vi "AO tester.vi"() -> ()   [LabVIEW 2013]
uses:
  Controls/FPGA Nain State.ctl
  <vilib>/Platform/TimedLoop/XDataNode/timing_clust.ctl
  <vilib>/Platform/TimedLoop/XDataNode/nitl_modes.ctl
  <vilib>/Platform/TimedLoop/XDataNode/wakeup.ctl
  Controls/Algorithm State.ctl
  <vilib>/rvi/Emulation/niFpgaSctlEmulationGetInTimedLoop.vi
  <vilib>/rvi/Emulation/niFpgaEmulationReportErrorSimple.vi
  <vilib>/rvi/Emulation/niFpgaGetClockAttributes.vi
  <vilib>/rvi/Emulation/niFpgaCriticalErrorInLSC.vi
  <vilib>/rvi/FIFO/Fifo_Resource/nirvififoEmulationReadFpgaImpl.vi
  <vilib>/rvi/DataTransferAndStorage/Container/Common/niFpgaContainerGetUniqueNameForEmu.vi
  <vilib>/rvi/interface/RandomDataEmulation/nirviRandomDataFPGAFIFO.vi
  <vilib>/rvi/interface/RandomDataEmulation/niFpgaRandomDataHandleErrors.vi
  <vilib>/rvi/eio/common/nirviEmuTemplateMethod_errors.vi
  <vilib>/rvi/FIFO/Fifo_Resource/nirvififoEmulationWriteFpgaImpl.vi
  LIDAR V2 Globals.vi
  <vilib>/rvi/Emulation/niFpgaProcessEmulError.vi
  <vilib>/Platform/TimedLoop/XDataNode/XDataNode.xnode
  <vilib>/rvi/DataTransferAndStorage/Container/XNode/niFpgaContainer.xnode
  <vilib>/rvi/FIFO/Fifo_Resource/nirvififoEmulationRead.vi
  <vilib>/rvi/interface/RandomDataEmulation/nirviRandomDataFpgaReadWriteTemplate.vi
  <vilib>/eio/EIONode/EIONode.xnode
  <vilib>/rvi/FIFO/Fifo_Resource/nirvififoEmulationWrite.vi
  <vilib>/Platform/TimedLoop/XDataNode/XDNodeRunTimeDep.lvlib
panel:
  out "EndOfPulseGen":bool
  in  "SingleFrame":bool
  out "Port1":u8 format="%.0b"
  out "Port1Bit5":bool
  out "Port1Bit4":bool
  out "Port0":u8 format="%.0b"
  in  "PFI2":bool
  in  "PFI3":bool
  in  "WaitForPulseEndDelay":u8=3
  in  "ActiveLedIndexDeb":u16
  in  "LedScanDebEn":bool
  in  "NoOfLeds":u16=320
  out "LedAddress":u16
  in  "SamplingEnable":bool
  out "MainState":T1
  in  "PulseEndClck":u8=3
  in  "PulseWaitClck":u8=40
  out "SimOut":i16
  out "PulseIndex":i16
  in  "PulsePerLed":i16=199
  in  "MemSel":bool
  out "ActiveLedIndex":u16
  in  "SampPerPulse":u8=100
  out "PulseEnd":bool
  out "Timeouts":u16
  in  "SPI Device":u8
  out "AI":i16
  in  "EnAI":bool
  in  "User Command Commit":bool
  in  "User Command":u8
  out "User Command Idle":bool
  out "User Command Status":u8
  in  "User Data 0":u8
  in  "User Data 1":u8
  out "User Error":bool
  out "Configured?":bool
  out "PLL Locked":bool
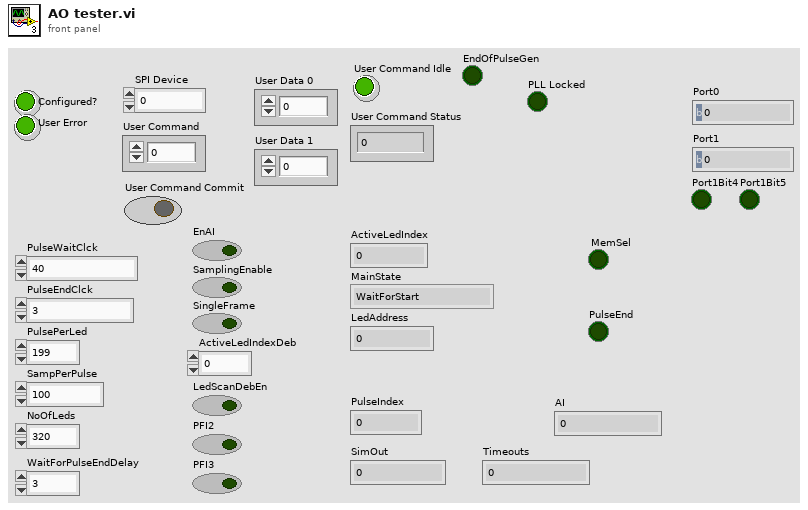
[diagram p1: front panel]
types:
  T1 = typedef "FPGA Nain State.ctl" = enum16{"WaitForStart", "SetProcParams", "SelectActiveLed", "WaitForPulseGenEnd", "ActivatePulse", "WaitForPulseEnd", "WaitForAlgoStart", "SingleCycleEnd"}
  T2 = typedef "XDNodeRunTimeDep.lvlib/timing_clust.ctl" = cluster{"Expected End [f-1]":u64, "Actual End [f-1]":u64, "Finished Late? [f-1]":bool, "Expected End [i-1]":u64, "Actual End [i-1]":u64, "Finished Late? [i-1]":bool, "Expected Start [i]":u64, "Actual Start [i]":u64, "Expected Start [f]":u64, "Actual Start [f]":u64, "Source Name":string, "Structure Name":string, "Period":i64, "Deadline":i64, "Offset":i64, "Start":i64, "Priority":i32, "Timeout":i32, "Mode":T3, "Wakeup Reason":T4, "Error":errorcluster, "Source Type":string, "Secondary Source Type":string, "Global End Time":u64, "Global Start Time":u64, "Frame Duration":u64, "Iteration Duration":u64, "Assigned CPU":i32, "I/O Scan Engine Mode":u32}
  T3 = typedef "XDNodeRunTimeDep.lvlib/nitl_modes.ctl" = enum32{"No Change", "Process missed periods, maintain original phase", "Discard missed periods, maintain original phase", "Process missed periods, ignore original phase", "Discard missed periods, ignore original phase"}
  T4 = typedef "XDNodeRunTimeDep.lvlib/wakeup.ctl" = enum32{"Normal", "Aborted", "Asynchronous wakeup", "Timing source error", "Timed loop error", "Timeout"}
  T5 = typedef "Algorithm State.ctl" = enum16{"WaitForStart", "GetNextSignalElement", "WaitForNextSignalElem", "MultWithSinc", "CalcMax"}
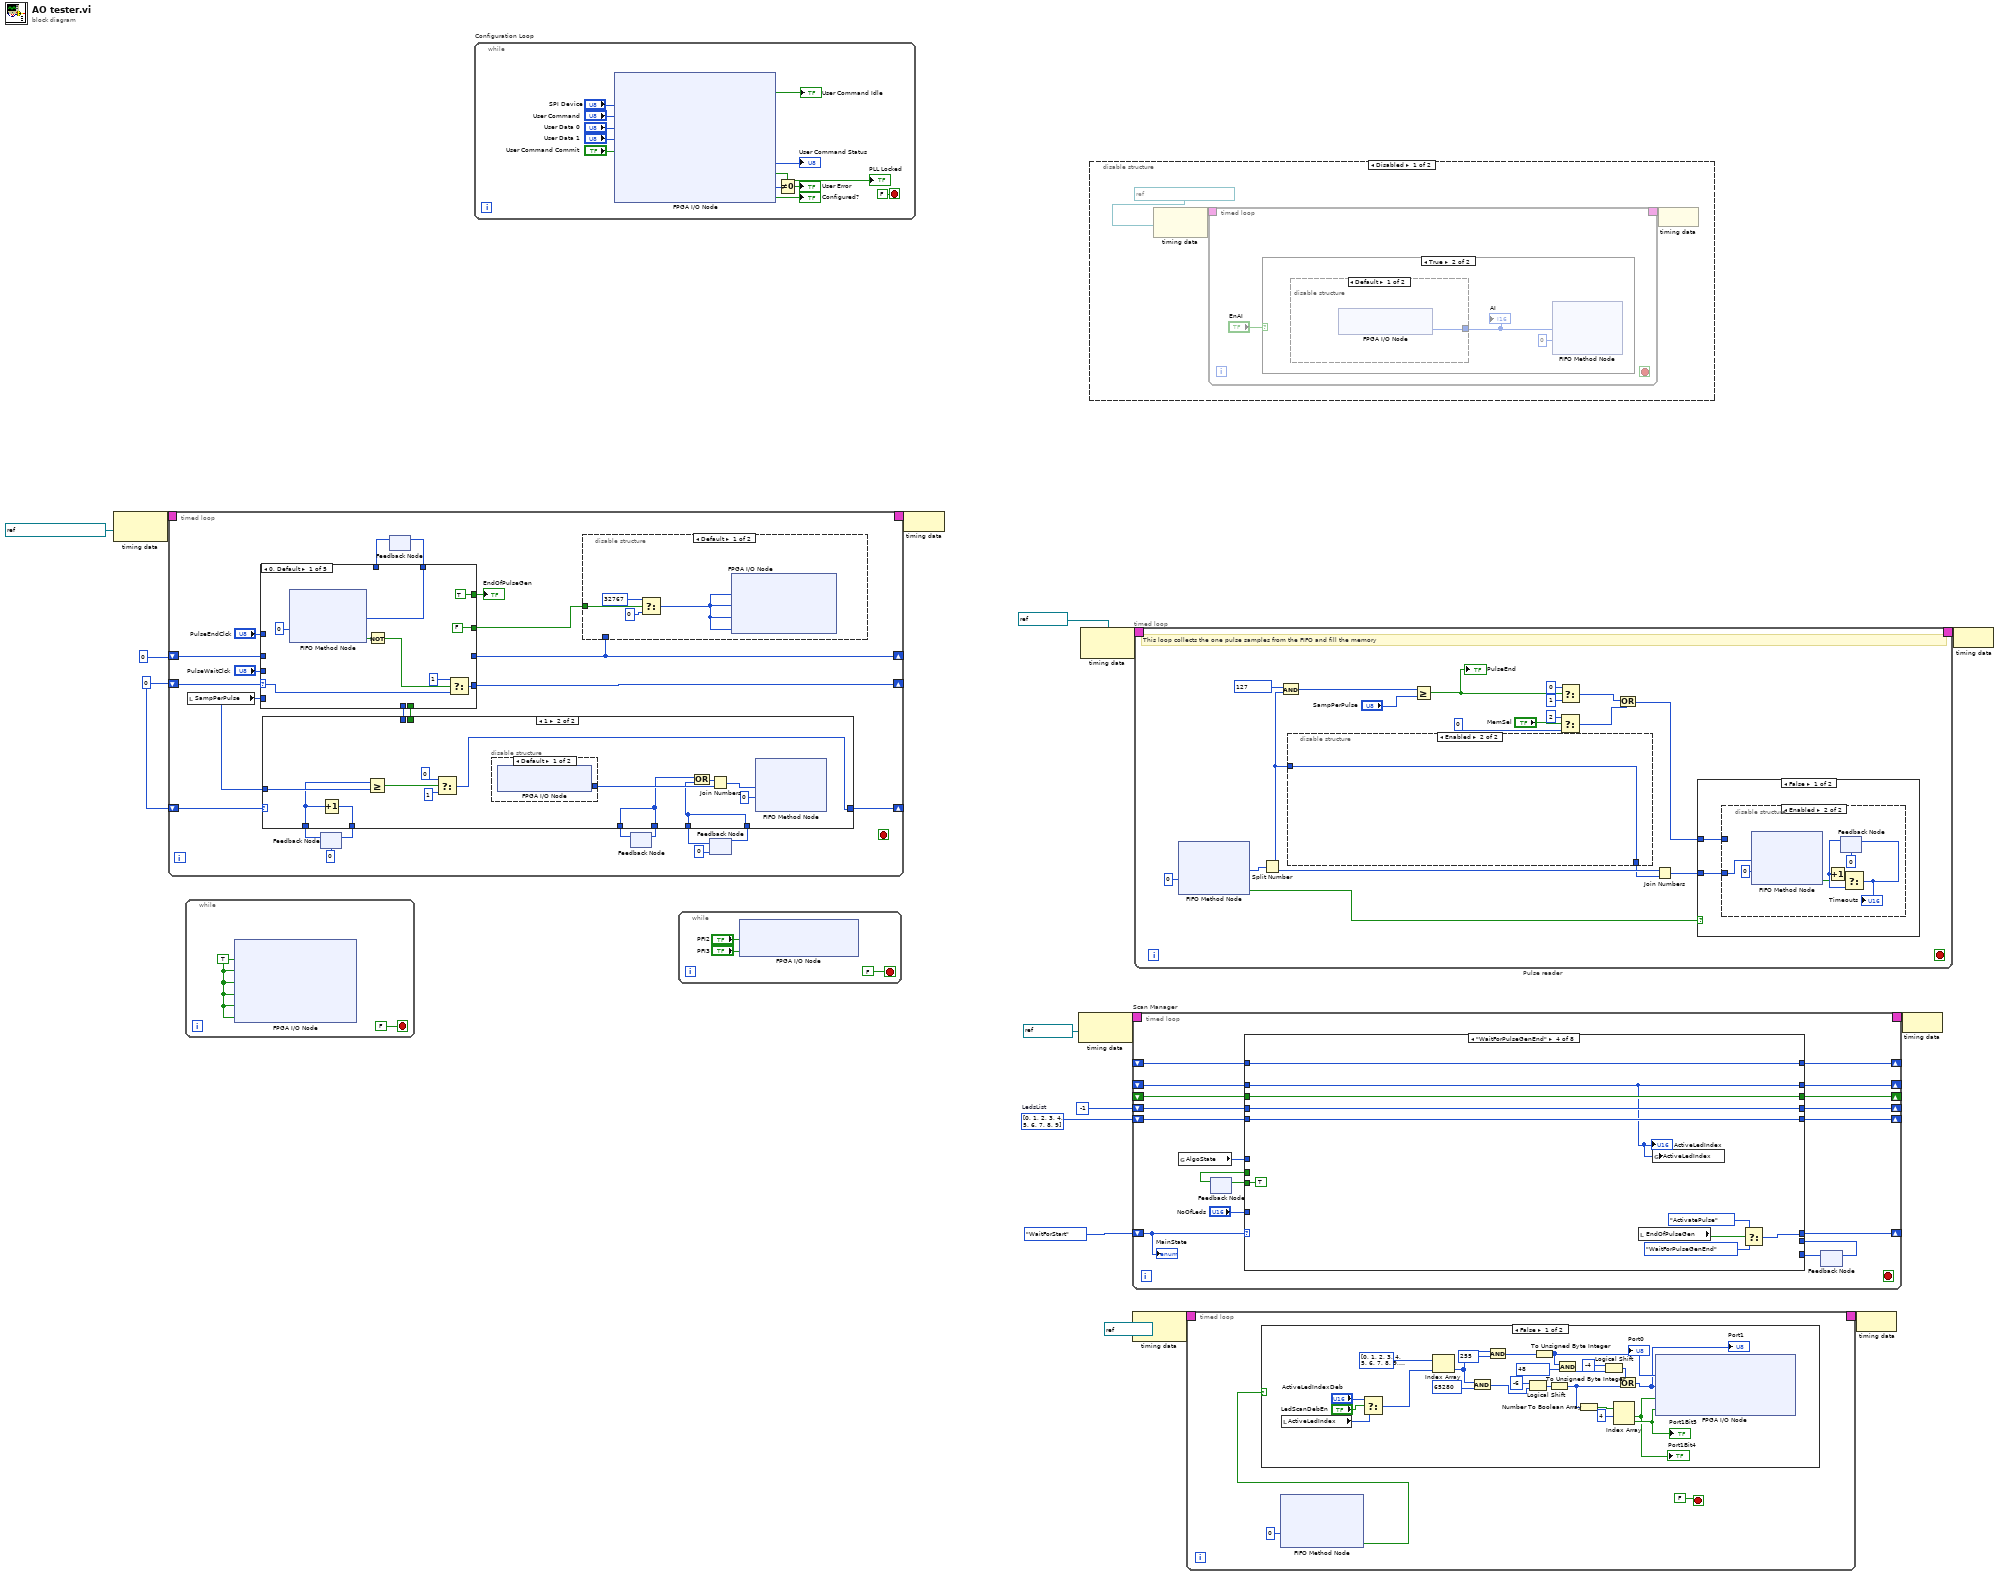
[diagram p0: block diagram]
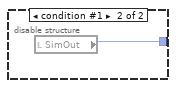
[diagram p3: hidden frame]
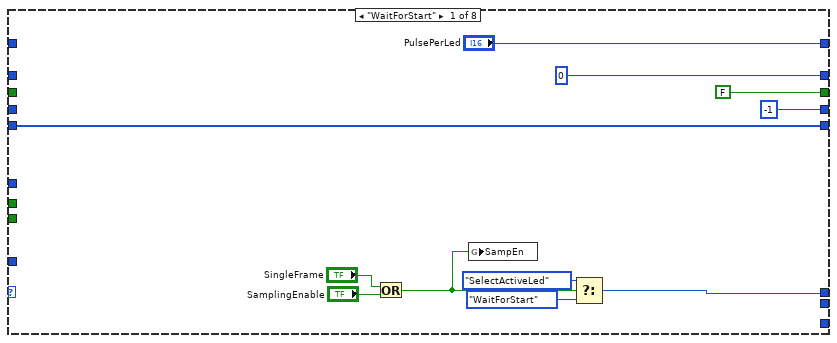
[diagram p6: hidden frame]
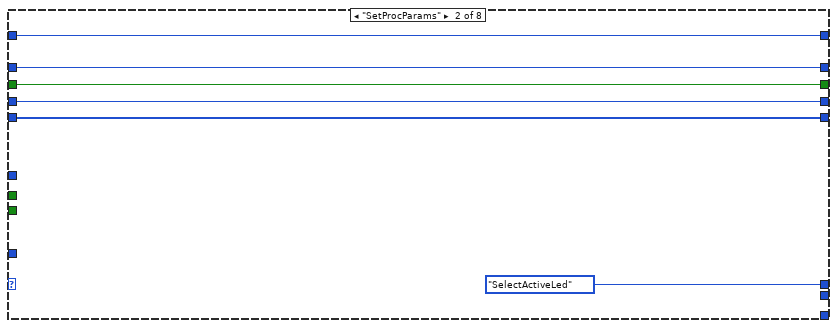
[diagram p7: hidden frame]
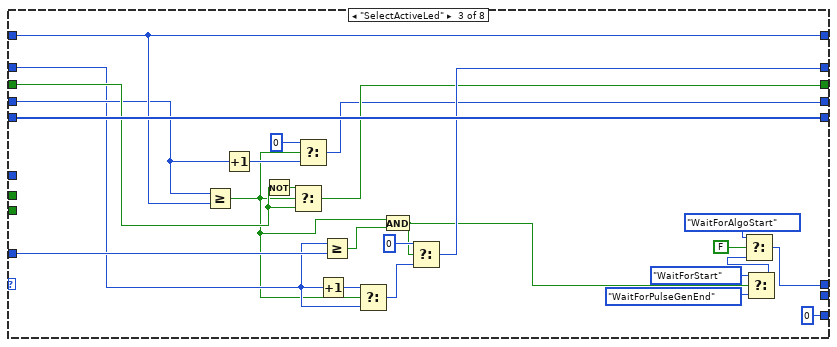
[diagram p8: hidden frame]
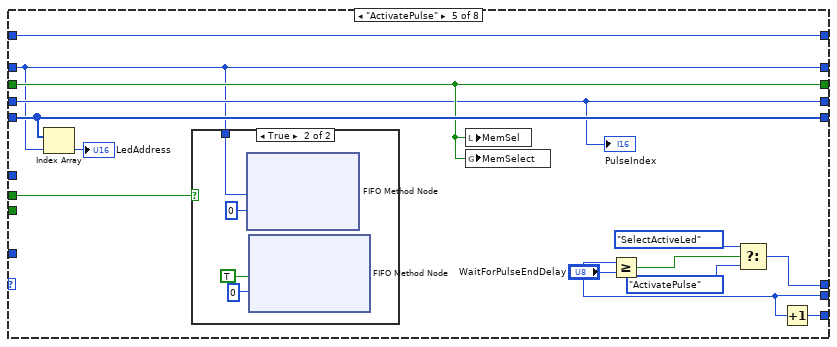
[diagram p9: hidden frame]
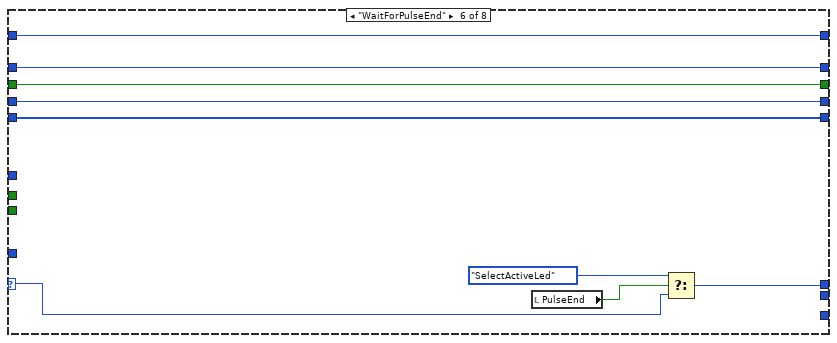
[diagram p11: hidden frame]
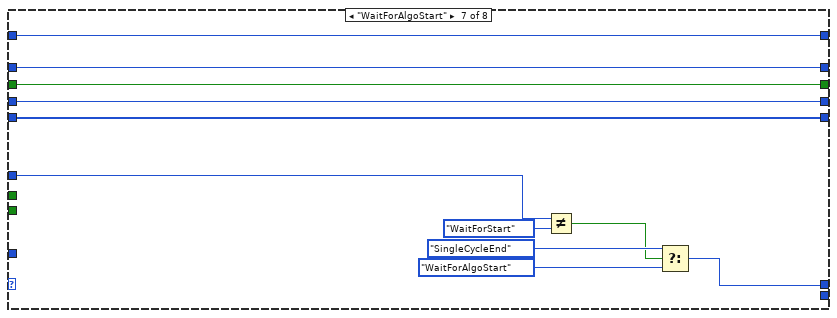
[diagram p12: hidden frame]
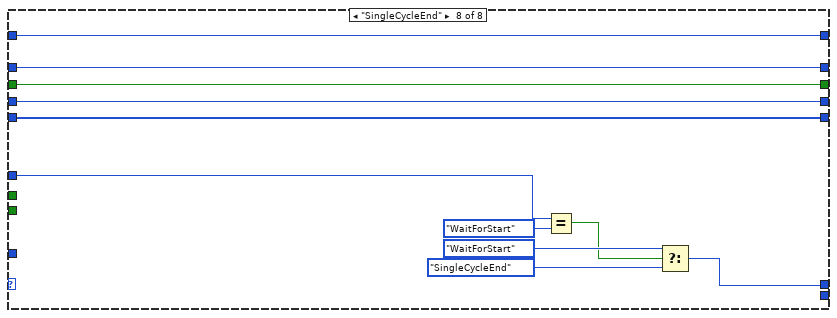
[diagram p13: hidden frame]
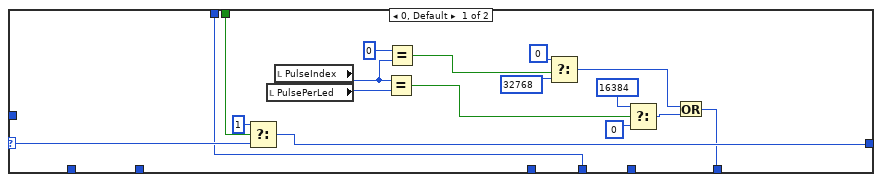
[diagram p14: hidden frame]
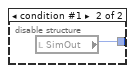
[diagram p15: hidden frame]
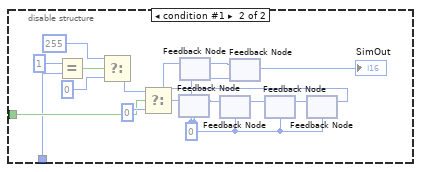
[diagram p16: hidden frame]
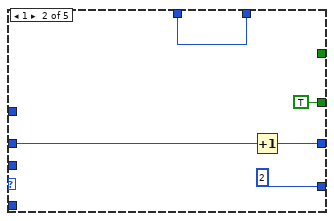
[diagram p17: hidden frame]
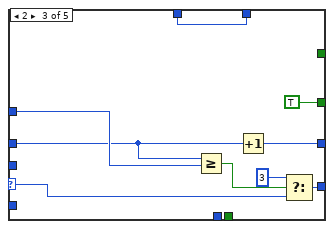
[diagram p18: hidden frame]
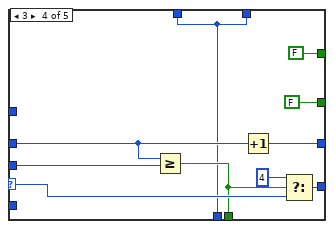
[diagram p19: hidden frame]
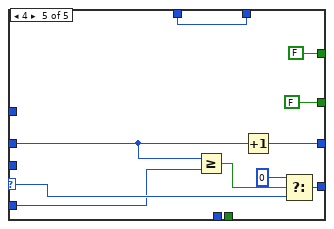
[diagram p20: hidden frame]
diagram:
  w6 = u16[] [0, 1, 2, 3, 4, 5, 6, 7, 8, 9]  # LedsList
  w1 = u8 0
  n1 = node-c288(refnum<k21> "IO Module\\Data Clock" ("Source Name")) -> (w14:T2)
  n2 = timed-loop {
    timing: w14 -> [_]
    timing-out: [_] -> w13
    shift-right: [w39] -> _
    shift-left: w1 -> [w40]
    shift-right: [w37] -> _
    shift-left: u8 0 -> [w38]
    shift-right: [w29] -> _
    shift-left: w1 -> [w31]
    stop <- _ stop-if-true
    n3 = local read "SampPerPulse"() -> (w20:u8)
    n4 = feedback #1(u8 0) -> (w22:u8)
    n5 = feedback #2() -> (w27:u16)  [unwired: 1 in]
    n6 = case shown="0, Default" w40 {
      selector: w40 -> [w95 _ w114 w124 w134]
      tunnel: [w101 u8 2 ("t") w115 w125 w135] -> w39
      tunnel: w38 -> [_ w105 w108 w120 w129]
      tunnel: [_ w106 w109 w121 w130] -> w37
      tunnel: [FALSE TRUE TRUE FALSE FALSE] -> w36
      tunnel: "PulseEndClck" -> [_ _ w111 _ _]
      tunnel: "PulseWaitClck" -> [_ _ _ w118 _]
      tunnel: w20 -> [_ _ _ _ w126]
      tunnel: [TRUE _ _ FALSE FALSE] -> w32
      tunnel: [_ _ _ w117 _] -> w30
      tunnel: [w93 w104 w107 w116 w127] -> w28
      tunnel: w27 -> [_ w104 w107 w116 w127]
      tunnel: [_ _ _ w116 _] -> w26
      frame 0, Default {
        n7 = xnode ("FIFO Method Node")("Timeout"=0) -> ("Element"=w93:u16, "Timed Out?"=w99:bool)  [unwired: 1 in, 1 out]
        n8 = Not(x=w99) -> (.not. x?=w97:bool)
        n9 = Select(t=u8 1, s=w97, f=w95) -> (s? t:f=w101:u8)
      }
      frame 1 {
        n10 = Increment(x=w105) -> (x+1=w106:u8)
      }
      frame 2 {
        n11 = Greater Or Equal?(x=w108, y=w111) -> (x >= y?=w110:bool)
        n12 = Increment(x=w108) -> (x+1=w109:u8)
        n13 = Select(t=u8 3, s=w110, f=w114) -> (s? t:f=w115:u8)
      }
      frame 3 {
        n14 = Greater Or Equal?(x=w120, y=w118) -> (x >= y?=w117:bool)
        n15 = Increment(x=w120) -> (x+1=w121:u8)
        n16 = Select(t=u8 4, s=w117, f=w124) -> (s? t:f=w125:u8)
      }
      frame 4 {
        n17 = Greater Or Equal?(x=w129, y=w126) -> (x >= y?=w131:bool)
        n18 = Increment(x=w129) -> (x+1=w130:u8)
        n19 = Select(t=u8 0, s=w131, f=w134) -> (s? t:f=w135:u8)
      }
    }
    "EndOfPulseGen" <- w32
    n20 = feedback-in #2(w28) -> ()
    n21 = disable-structure shown="Default" {
      disable-tunnel: w36 -> [w73 w84]
      disable-tunnel: w37 -> [_ w83]
      frame condition #0 (active) {
        n22 = Select(t=i16 32767 ("IO Module\\AO 0 N"), s=w73, f=i16 0) -> (s? t:f=w74:i16)
        n23 = xnode "FPGA I/O Node"("IO Module\\AO 0 N-3"=w74, "IO Module\\AO 0 N-2"=w74, "IO Module\\AO 0 N-1"=w74, "IO Module\\AO 0 N"=w74) -> ()  [unwired: 4 in, 4 out]
      }
      frame condition #1 {
        w87 = i16 0 ("IO Module\\AO 0")
        n24 = Equal?(x=u16 1, y=w83) -> (x = y?=w81:bool)
        n25 = Select(t=i16 255 ("IO Module\\AO 0"), s=w81, f=i16 0) -> (s? t:f=w82:i16)
        n26 = Select(t=w82, s=w84, f=i16 0 ("IO Module\\AO 0")) -> (s? t:f=w85:i16)
        n27 = feedback-in #3(w85) -> ()
        n28 = feedback #3(w87) -> (w92:i16)
        n29 = feedback #4(w87) -> (w88:i16)
        n30 = feedback #5(w87) -> (w91:i16)
        n31 = feedback-in #5(w92) -> ()
        n32 = feedback #6(w87) -> (→"SimOut":i16)
        n33 = feedback-in #6(w88) -> ()
        n34 = feedback #7(w87) -> (w90:i16)
        n35 = feedback-in #7(w91) -> ()
        n36 = feedback #8(w87) -> (w89:i16)
        n37 = feedback-in #4(w89) -> ()
        n38 = feedback-in #8(w90) -> ()
      }
    }
    n39 = feedback #9() -> (w25:u16)  [unwired: 1 in]
    n40 = feedback #10(u16 0) -> (w18:u16)
    n41 = case shown="1" w31 {
      selector: w31 -> [w56 _]
      tunnel: w30 -> [w57 _]
      tunnel: [w54 w61] -> w29
      tunnel: [w53 w59] -> w24
      tunnel: w26 -> [w53 _]
      tunnel: w25 -> [_ w59]
      tunnel: w22 -> [_ w60]
      tunnel: [_ w70] -> w21
      tunnel: w20 -> [_ w69]
      tunnel: [w41 w58] -> w19
      tunnel: w18 -> [_ w58]
      frame 0, Default {
        n42 = Select(t=u8 1, s=w57, f=w56) -> (s? t:f=w54:u8)
        n43 = local read "PulsePerLed"() -> (w51:i16)
        n44 = local read "PulseIndex"() -> (w52:i16)
        n45 = Equal?(x=w52, y=w51) -> (x = y?=w46:bool)
        n46 = Equal?(x=i16 0, y=w52) -> (x = y?=w44:bool)
        n47 = Select(t=u16 0 ("x"), s=w44, f=u16 32768 ("FirstIterration")) -> (s? t:f=w42:u16)
        n48 = Select(t=u16 16384 ("LastIterration"), s=w46, f=u16 0 ("x")) -> (s? t:f=w43:u16)
        n49 = Or(x=w42, y=w43) -> (x .or. y?=w41:u16)
      }
      frame 1 {
        n50 = Increment(x=w60) -> (x+1=w70:u8)
        n51 = Greater Or Equal?(x=w60, y=w69) -> (x >= y?=w68:bool)
        n52 = Select(t=u8 0, s=w68, f=u8 1) -> (s? t:f=w61:u8)
        n53 = disable-structure shown="Default" {
          disable-tunnel: [w71 w72] -> w63
          frame condition #0 (active) {
            n54 = xnode "FPGA I/O Node"() -> ("IO Module\\AI 0 N"=w71:i16)  [unwired: 1 in, 1 out]
          }
          frame condition #1 {
            n55 = local read "SimOut"() -> (w72:i16)
          }
        }
        n56 = Or(x=w59, y=w58) -> (x .or. y?=w65:u16)
        n57 = Join Numbers(hi=w65, lo=w63) -> ((hi.lo)=w64:u32)
        n58 = xnode ("FIFO Method Node")("Element"=w64, "Timeout"=0) -> ()  [unwired: 1 in, 2 out]
      }
    }
    n59 = feedback-in #1(w21) -> ()
    n60 = feedback-in #9(w24) -> ()
    n61 = feedback-in #10(w19) -> ()
  }
  n62 = while {
    stop <- FALSE stop-if-true
    w138 = TRUE ("IO Module\\DIO Port 0 WE")
    n63 = xnode "FPGA I/O Node"("IO Module\\DIO Port 0 WE"=w138, "IO Module\\DIO Port 1 WE"=w138, "IO Module\\PFI 0 WE"=w138, "IO Module\\PFI 1 WE"=w138, "IO Module\\PFI 2 WE"=w138, "IO Module\\PFI 3 WE"=w138) -> ()  [unwired: 6 in, 6 out]
  }
  n64 = while "Configuration Loop" {
    stop <- FALSE stop-if-true
    n65 = xnode "FPGA I/O Node"("IO Module\\SPI Device"="SPI Device", "IO Module\\User Command"="User Command", "IO Module\\User Data 0"="User Data 0", "IO Module\\User Data 1"="User Data 1", "IO Module\\User Command Commit"="User Command Commit") -> ("IO Module\\User Command Idle"=→"User Command Idle":bool, "IO Module\\User Command Status"=→"User Command Status":u8, "IO Module\\PLL Locked"=→"PLL Locked":bool, "IO Module\\User Error"=w145:u8, "IO Module\\Initialization Done"=→"Configured?":bool)  [unwired: 10 in, 10 out]
    n66 = Not Equal To 0?(x=w145) -> (x != 0?=→"User Error":bool)
  }
  n67 = while {
    stop <- FALSE stop-if-true
    n68 = xnode "FPGA I/O Node"("IO Module\\PFI 2 Wr Data"="PFI2", "IO Module\\PFI 3 Wr Data"="PFI3") -> ()  [unwired: 2 in, 2 out]
  }
  n69 = node-c288(w13) -> ()
  n70 = node-c288(refnum<k21> "130MHz" ("Source Name")) -> (w10:T2)
  n71 = node-c288(refnum<k21> "130MHz" ("Source Name")) -> (w17:T2)
  n72 = disable-structure shown="Disabled" {
    frame Disabled {
      n73 = node-c288(refnum<k21> "IO Module\\Data Clock" ("Source Name")) -> (w157:T2)
      n74 = timed-loop {
        timing: w157 -> [_]
        timing-out: [_] -> w156
        stop <- _ stop-if-true
        n75 = case shown="True" "EnAI" {
          frame False {
          }
          frame True {
            n76 = disable-structure shown="Default" {
              disable-tunnel: [w161 w162] -> w159
              frame condition #0 (active) {
                n77 = xnode "FPGA I/O Node"() -> ("IO Module\\AI 0 N"=w161:i16)  [unwired: 1 in, 1 out]
              }
              frame condition #1 {
                n78 = local read "SimOut"() -> (w162:i16)
              }
            }
            "AI" <- w159
            n79 = xnode ("FIFO Method Node")("Element"=w159, "Timeout"=0) -> ()  [unwired: 1 in, 2 out]
          }
        }
      }
      n80 = node-c288(w156) -> ()
    }
    frame Enabled {
    }
  }
  n81 = node-c288(refnum<k21> "130MHz" ("Source Name")) -> (w4:T2)
  n82 = timed-loop "Scan Manager" {
    timing: w10 -> [_]
    timing-out: [_] -> w9
    shift-right: [w185] -> _
    shift-left: FPGA_Nain_State."WaitForStart" ("MainState") -> [w186]
    shift-right: [w184] -> _
    shift-left: _ -> [w183]
    shift-right: [w173] -> _
    shift-left: _ -> [w182]
    shift-right: [w177] -> _
    shift-left: _ -> [w181]
    shift-right: [w180] -> _
    shift-left: i16 -1 -> [w176]
    shift-right: [w178] -> _
    shift-left: w6 -> [w179]
    stop <- _ stop-if-true
    n83 = global read "LIDAR V2 Globals.vi" "AlgoState"() -> (w172:T5)
    n84 = feedback #11() -> (w174:bool)  [unwired: 1 in]
    n85 = feedback #12() -> (w169:u8)  [unwired: 1 in]
    n86 = case shown="\"WaitForPulseGenEnd\"" w186 {
      selector: w186 -> [_ _ _ _ _ w262 _ _]
      tunnel: [w195 FPGA_Nain_State."SelectActiveLed" ("MainState") w224 w231 w240 w261 w269 w280] -> w185
      tunnel: ["PulsePerLed" w200 w222 w238 w252 w265 w276 w287] -> w184
      tunnel: w183 -> [_ w200 w222 w238 w252 w265 w276 w287]
      tunnel: [u16 0 ("ActiveLedIndex") w199 w219 w230 w239 w264 w275 w286] -> w173
      tunnel: w182 -> [_ w199 w211 w230 w239 w264 w275 w286]
      tunnel: [FALSE w198 w218 w237 w248 w263 w274 w285] -> w177
      tunnel: w181 -> [_ w198 w221 w237 w248 w263 w274 w285]
      tunnel: [i16 -1 ("t") w202 w214 w236 w247 w259 w273 w284] -> w180
      tunnel: w176 -> [_ w202 w217 w236 w247 w259 w273 w284]
      tunnel: w179 -> [w193 w201 w228 w235 w249 w258 w272 w283]
      tunnel: [w193 w201 w228 w235 w249 w258 w272 w283] -> w178
      tunnel: [_ _ _ TRUE _ _ _ _] -> w175
      tunnel: w174 -> [_ _ _ _ w251 _ _ _]
      tunnel: w172 -> [_ _ _ _ _ _ w266 w278]
      tunnel: "NoOfLeds" -> [_ _ w213 _ _ _ _ _]
      tunnel: [_ _ u8 0 _ w246 _ _ _] -> w170
      tunnel: w169 -> [_ _ _ _ w245 _ _ _]
      frame "WaitForStart" {
        n87 = Or(x="SingleFrame", y="SamplingEnable") -> (x .or. y?=w188:bool)
        n88 = global write "LIDAR V2 Globals.vi" "SampEn"(w188) -> ()
        n89 = Select(t=FPGA_Nain_State."SelectActiveLed" ("MainState"), s=w188, f=FPGA_Nain_State."WaitForStart" ("MainState")) -> (s? t:f=w195:T1)
      }
      frame "SetProcParams" {
      }
      frame "SelectActiveLed" {
        n90 = Greater Or Equal?(x=w217, y=w222) -> (x >= y?=w206:bool)
        n91 = Increment(x=w217) -> (x+1=w216:i16)
        n92 = Not(x=w221) -> (.not. x?=w220:bool)
        n93 = Select(t=w220, s=w206, f=w221) -> (s? t:f=w218:bool)
        n94 = Select(t=i16 0, s=w206, f=w216) -> (s? t:f=w214:i16)
        n95 = Increment(x=w211) -> (x+1=w209:u16)
        n96 = Greater Or Equal?(x=w211, y=w213) -> (x >= y?=w207:bool)
        n97 = Select(t=w209, s=w206, f=w211) -> (s? t:f=w210:u16)
        n98 = And(x=w206, y=w207) -> (x .and. y?=w205:bool)
        n99 = Select(t=u16 0, s=w205, f=w210) -> (s? t:f=w219:u16)
        n100 = Select(t=FPGA_Nain_State."WaitForStart" ("MainState"), s=w205, f=FPGA_Nain_State."WaitForPulseGenEnd" ("MainState")) -> (s? t:f=w225:T1)
        n101 = Select(t=FPGA_Nain_State."WaitForAlgoStart" ("MainState"), s=FALSE, f=w225) -> (s? t:f=w224:T1)
      }
      frame "WaitForPulseGenEnd" {
        n102 = local read "EndOfPulseGen"() -> (w234:bool)
        n103 = global write "LIDAR V2 Globals.vi" "ActiveLedIndex"(w230) -> ()
        n104 = Select(t=FPGA_Nain_State."ActivatePulse" ("MainState"), s=w234, f=FPGA_Nain_State."WaitForPulseGenEnd" ("MainState")) -> (s? t:f=w231:T1)
        "ActiveLedIndex" <- w230
      }
      frame "ActivatePulse" {
        n105 = Index Array(array=w249, index=w239) -> (element=→"LedAddress":u16)
        n106 = case shown="True" w251 {
          tunnel: w239 -> [_ w253]
          frame False {
          }
          frame True {
            n107 = xnode ("FIFO Method Node")("Element"=w253, "Timeout"=0) -> ()  [unwired: 1 in, 2 out]
            n108 = xnode ("FIFO Method Node")("Element"=TRUE ("GenPulse"), "Timeout"=0) -> ()  [unwired: 1 in, 2 out]
          }
        }
        n109 = local write "MemSel"(w248) -> ()
        n110 = global write "LIDAR V2 Globals.vi" "MemSelect"(w248) -> ()
        n111 = Greater Or Equal?(x=w245, y="WaitForPulseEndDelay") -> (x >= y?=w243:bool)
        n112 = Select(t=FPGA_Nain_State."SelectActiveLed" ("MainState"), s=w243, f=FPGA_Nain_State."ActivatePulse" ("MainState")) -> (s? t:f=w240:T1)
        n113 = Increment(x=w245) -> (x+1=w246:u8)
        "PulseIndex" <- w247
      }
      frame "WaitForPulseEnd" {
        n114 = local read "PulseEnd"() -> (w257:bool)
        n115 = Select(t=FPGA_Nain_State."SelectActiveLed", s=w257, f=w262) -> (s? t:f=w261:T1)
      }
      frame "WaitForAlgoStart" {
        n116 = Not Equal?(x=w266, y=Algorithm_State."WaitForStart") -> (x != y?=w267:bool)
        n117 = Select(t=FPGA_Nain_State."SingleCycleEnd", s=w267, f=FPGA_Nain_State."WaitForAlgoStart" ("MainState")) -> (s? t:f=w269:T1)
      }
      frame "SingleCycleEnd" {
        n118 = Equal?(x=w278, y=Algorithm_State."WaitForStart") -> (x = y?=w277:bool)
        n119 = Select(t=FPGA_Nain_State."WaitForStart", s=w277, f=FPGA_Nain_State."SingleCycleEnd" ("MainState")) -> (s? t:f=w280:T1)
      }
    }
    n120 = feedback-in #11(w175) -> ()
    n121 = feedback-in #12(w170) -> ()
    "MainState" <- w186
  }
  n122 = timed-loop "Pulse reader" {
    timing: w17 -> [_]
    timing-out: [_] -> w16
    stop <- _ stop-if-true
    # "This loop collects the one pulse samples from the FIFO and fill the memory"
    n123 = xnode ("FIFO Method Node")("Timeout"=0) -> ("Element"=w304:u32, "Timed Out?"=w294:bool)  [unwired: 1 in, 1 out]
    n124 = Split Number(x=w304) -> (hi(x)=w291:u16, lo(x)=w303:u16)
    n125 = And(x=u16 127, y=w291) -> (x .and. y?=w293:u16)
    n126 = disable-structure shown="Enabled" {
      disable-tunnel: [w316 w325] -> w295
      disable-tunnel: w291 -> [w312 w325]
      frame Disabled {
        w321 = u16 16384  # LastIterration
        w318 = u16 32768  # FirstIterration
        n127 = local read "PulsePerLed"() -> (w323:i16)
        n128 = Logical Shift(y=i16 -7, x=w312) -> (x << y=w309:u16)
        n129 = local read "PulseIndex"() -> (w324:i16)
        n130 = Equal?(x=w324, y=w323) -> (x = y?=w315:bool)
        n131 = Equal?(x=i16 0, y=w324) -> (x = y?=w313:bool)
        n132 = Select(t=u16 0 ("x"), s=w313, f=w318) -> (s? t:f=w310:u16)
        n133 = Select(t=w321, s=w315, f=u16 0 ("x")) -> (s? t:f=w320:u16)
        n134 = Or(x=w309, y=w310) -> (x .or. y?=w319:u16)
        n135 = Or(x=w319, y=w320) -> (x .or. y?=w316:u16)
      }
      frame Enabled {
      }
    }
    n136 = Greater Or Equal?(x=w293, y="SampPerPulse") -> (x >= y?=w305:bool)
    "PulseEnd" <- w305
    n137 = Select(t=i16 2, s="MemSel", f=i16 0) -> (s? t:f=w297:i16)
    n138 = Select(t=i16 0, s=w305, f=i16 1) -> (s? t:f=w296:i16)
    n139 = Or(x=w296, y=w297) -> (x .or. y?=w298:i16)
    n140 = Join Numbers(hi=w303, lo=w295) -> ((hi.lo)=w302:u32)
    n141 = case shown="False" w294 {
      tunnel: w302 -> [w327 _]
      tunnel: w298 -> [w326 _]
      frame False {
        n142 = disable-structure shown="Enabled" {
          disable-tunnel: w327 -> [w329 w330]
          disable-tunnel: w326 -> [w328 _]
          frame Disabled {
            n143 = case shown="1" w328 {
              tunnel: w329 -> [_ _ _]
              frame 1 {
                (unwired) 0 ("Timeout")
                n144 = xnode ("FIFO Method Node")() -> ()  [unwired: 3 in, 2 out]
              }
              frame 3 {
                (unwired) 0 ("Timeout")
                n145 = xnode ("FIFO Method Node")() -> ()  [unwired: 3 in, 2 out]
              }
              frame Default {
              }
            }
          }
          frame Enabled {
            n146 = xnode ("FIFO Method Node")("Element"=w330, "Timeout"=0) -> ("Timed Out?"=w332:bool)  [unwired: 1 in, 1 out]
            n147 = feedback #13(u16 0) -> (w335:u16)
            n148 = Increment(x=w335) -> (x+1=w336:u16)
            n149 = Select(t=w336, s=w332, f=w335) -> (s? t:f=w334:u16)
            "Timeouts" <- w334
            n150 = feedback-in #13(w334) -> ()
          }
        }
      }
      frame True {
      }
    }
  }
  n151 = timed-loop {
    timing: w4 -> [_]
    timing-out: [_] -> w3
    stop <- FALSE stop-if-true
    n152 = xnode ("FIFO Method Node")("Timeout"=0) -> ("Timed Out?"=w339:bool)  [unwired: 1 in, 2 out]
    n153 = case shown="False" w339 {
      frame False {
        n154 = local read "ActiveLedIndex"() -> (w360:u16)
        n155 = Select(t="ActiveLedIndexDeb", s="LedScanDebEn", f=w360) -> (s? t:f=w353:u16)
        n156 = Index Array(array=u16[] [0, 1, 2, 3, 4, 5, 6, 7, 8, 9, 10, 11, 12, 13, 14, 15, 16, 17, 18, 19, 256, 257, 258, 259, 260, 261, 262, 263, 264, 265, 266, 267, 268, 269, 270, 271, 272, 273, 274, 275, 512, 513, 514, 515, 516, 517, 518, 519, 520, 521, 522, 523, 524, 525, 526, 527, 528, 529, 530, 531, 768, 769, 770, 771, 772, 773, 774, 775, 776, 777, 778, 779, 780, 781, 782, 783, 784, 785, 786, 787, 1024, 1025, 1026, 1027, 1028, 1029, 1030, 1031, 1032, 1033, 1034, 1035, 1036, 1037, 1038, 1039, 1040, 1041, 1042, 1043, 1280, 1281, 1282, 1283, 1284, 1285, 1286, 1287, 1288, 1289, 1290, 1291, 1292, 1293, 1294, 1295, 1296, 1297, 1298, 1299, 1536, 1537, 1538, 1539, 1540, 1541, 1542, 1543, 1544, 1545, 1546, 1547, 1548, 1549, 1550, 1551, 1552, 1553, 1554, 1555, 1792, 1793, 1794, 1795, 1796, 1797, 1798, 1799, 1800, 1801, 1802, 1803, 1804, 1805, 1806, 1807, 1808, 1809, 1810, 1811, 2048, 2049, 2050, 2051, 2052, 2053, 2054, 2055, 2056, 2057, 2058, 2059, 2060, 2061, 2062, 2063, 2064, 2065, 2066, 2067, 2304, 2305, 2306, 2307, 2308, 2309, 2310, 2311, 2312, 2313, 2314, 2315, 2316, 2317, 2318, 2319, 2320, 2321, 2322, 2323, 2560, 2561, 2562, 2563, 2564, 2565, 2566, 2567, 2568, 2569, 2570, 2571, 2572, 2573, 2574, 2575, 2576, 2577, 2578, 2579, 2816, 2817, 2818, 2819, 2820, 2821, 2822, 2823, 2824, 2825, 2826, 2827, 2828, 2829, 2830, 2831, 2832, 2833, 2834, 2835, 3072, 3073, 3074, 3075, 3076, 3077, 3078, 3079, 3080, 3081, 3082, 3083, 3084, 3085, 3086, 3087, 3088, 3089, 3090, 3091, 3328, 3329, 3330, 3331, 3332, 3333, 3334, 3335, 3336, 3337, 3338, 3339, 3340, 3341, 3342, 3343, 3344, 3345, 3346, 3347, 3584, 3585, 3586, 3587, 3588, 3589, 3590, 3591, 3592, 3593, 3594, 3595, 3596, 3597, 3598, 3599, 3600, 3601, 3602, 3603, 3840, 3841, 3842, 3843, 3844, 3845, 3846, 3847, 3848, 3849, 3850, 3851, 3852, 3853, 3854, 3855, 3856, 3857, 3858, 3859] ("Array"), index=w353) -> (element=w356:u16)
        n157 = And(x=w356, y=u16 65280) -> (x .and. y?=w351:u16)
        n158 = And(x=w356, y=u16 255) -> (x .and. y?=w352:u16)
        n159 = Logical Shift(y=i16 -6, x=w351) -> (x << y=w350:u16)
        n160 = To Unsigned Byte Integer(number=w352) -> (unsigned 8bit integer=w348:u8)
        "Port0" <- w348
        n161 = To Unsigned Byte Integer(number=w350) -> (unsigned 8bit integer=w344:u8)
        n162 = And(x=w348, y=u8 48) -> (x .and. y?=w347:u8)
        n163 = Number To Boolean Array(number=w344) -> (Boolean array=w364:bool[])
        n164 = Logical Shift(y=i16 -4, x=w347) -> (x << y=w343:u8)
        n165 = Index Array(array=w364, index #1=4 ("index")) -> (element #1=w345:bool, element #2=w362:bool)  [unwired: 1 in]
        "Port1Bit4" <- w345
        "Port1Bit5" <- w362
        n166 = Or(x=w343, y=w344) -> (x .or. y?=w342:u8)
        "Port1" <- w342
        n167 = xnode "FPGA I/O Node"("IO Module\\DIO Port 0 Wr Data"=w348, "IO Module\\DIO Port 1 Wr Data"=w342, "IO Module\\PFI 0 Wr Data"=w345, "IO Module\\PFI 1 Wr Data"=w362) -> ()  [unwired: 4 in, 4 out]
      }
      frame True {
      }
    }
  }
  n168 = node-c288(w3) -> ()
  n169 = node-c288(w9) -> ()
  n170 = node-c288(w16) -> ()
